vi "2D Animation Plot.vi"(4 "sample length":i32=1000, 6 "angle unit":u16(ring) items=["radians", "degrees"], 7 "reset":bool, 9 "Goal":cluster{"x":dbl, "y":dbl}={"x"=nan, "y"=nan}, 10 "2D Origin":cluster{"x":dbl, "y":dbl, "theta":dbl}, 11 "2D Translation":cluster{"x":dbl, "y":dbl, "theta":dbl}) -> (3 "Coordinate Frame":cluster{dbl[], dbl[]}[](graph))   [LabVIEW 2017]
uses:
  <vilib>/Analysis/baseanly.llb/Real A x B.vi
  LabVIEW Corke Toolkit/Functions/Position and Orientation/rvc Plot 2D Transform (scalar).vi
  <vilib>/ptbypt/NI_PtbyPt.lvlib
  <vilib>/Analysis/NI_AALBase.lvlib
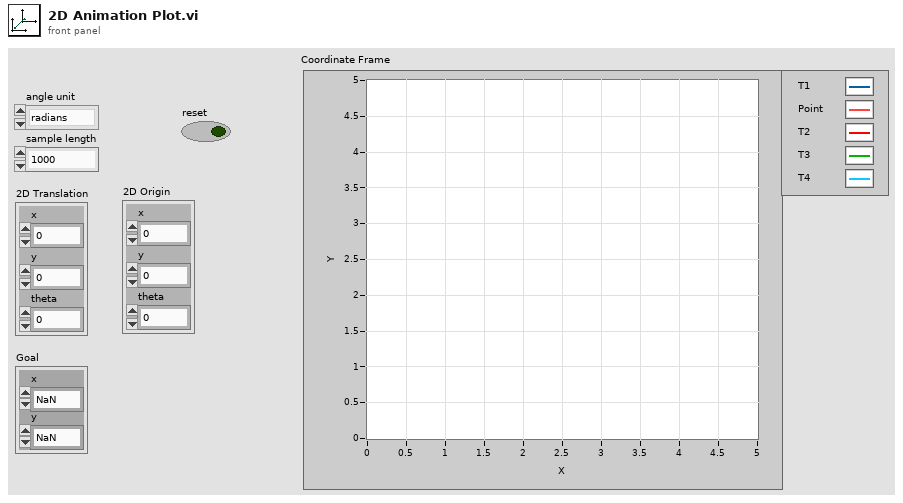
[diagram p1: front panel]
types:
  T1 = typedef "NI_Matrix.lvlib/RealMatrix.ctl" = dbl[][]
  T2 = cluster{"Current Queue":dbl[], "Current Queue":dbl[]}
  T3 = cluster{"Current Queue":dbl[], "Current Queue":dbl[]}[]
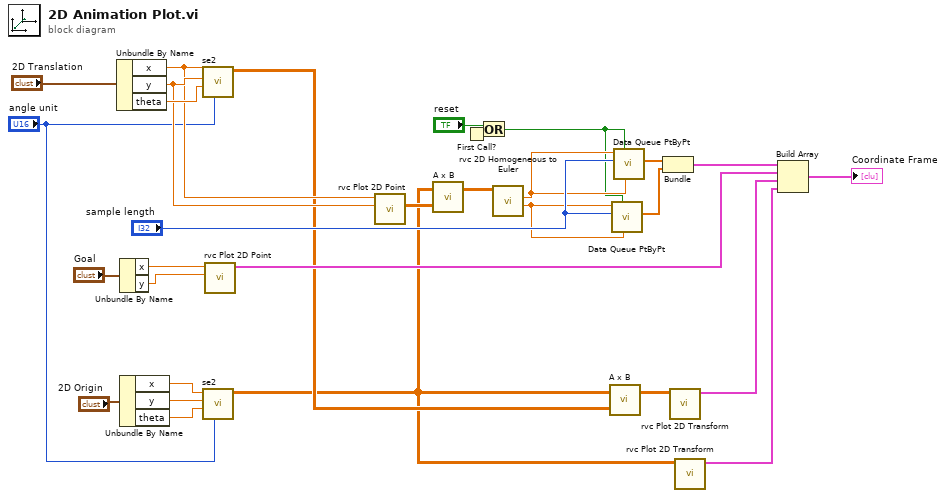
[diagram p0: block diagram]
diagram:
  n1 = Unbundle By Name("2D Translation") -> ("x"=w11:dbl, "y"=w12:dbl, "theta"=w25:dbl)
  n2 = Unbundle By Name("Goal") -> ("x"=w28:dbl, "y"=w27:dbl)
  n3 = Unbundle By Name("2D Origin") -> ("x"=w17:dbl, "y"=w16:dbl, "theta"=w15:dbl)
  n4 = call "se2.vi"("angle unit"="angle unit", "theta"=w25, "y"=w12, "x"=w11) -> ("T"=w10:dbl[][])  [unwired: 6 in, 1 out]
  n5 = call "se2.vi"("angle unit"="angle unit", "theta"=w15, "y"=w16, "x"=w17) -> ("T"=w8:dbl[][])  [unwired: 6 in, 1 out]
  n6 = call "rvc Plot 2D Point.vi"("Y"=w27, "X"=w28) -> ("XY Graph"=w30:cluster{dbl[], dbl[]})  [unwired: 8 in, 1 out]
  n7 = call "rvc Plot 2D Point.vi"("Y"=w12, "X"=w11) -> ("Column vector"=w9:dbl[][])  [unwired: 8 in, 1 out]
  n8 = call-poly <vilib>:"A x B.vi"("B"=w9, "A"=w8) -> ("A x B"=w13:T1)  [unwired: 1 out]
  n9 = First Call?() -> (First Call?: T/F=w5:bool)
  n10 = Or(x="reset", y=w5) -> (x .or. y?=w2:bool)
  n11 = call "rvc 2D Homogeneous to Euler.vi"("T"=w13) -> ("y"=w3:dbl, "x"=w4:dbl)  [unwired: 7 in, 2 out]
  n12 = call-poly <vilib>:"A x B.vi"("B"=w10, "A"=w8) -> ("A x B"=w14:T1)  [unwired: 1 out]
  n13 = call <vilib>:"Data Queue PtByPt.vi"("initial queue element"=w3, "initialize"=w2, "sample length"="sample length", "input data point"=w3) -> ("Current Queue"=w20:dbl[])  [unwired: 3 in, 4 out]
  n14 = call <vilib>:"Data Queue PtByPt.vi"("initial queue element"=w4, "initialize"=w2, "sample length"="sample length", "input data point"=w4) -> ("Current Queue"=w21:dbl[])  [unwired: 3 in, 4 out]
  n15 = Bundle("Current Queue"=w21, "Current Queue"=w20) -> (w19:T2)  [unwired: 1 in]
  n16 = call-poly "rvc Plot 2D Transform.vi"("T"=w14) -> ("XY Graph 2"=w24:cluster{dbl[], dbl[]})  [unwired: 9 in, 1 out]
  n17 = call-poly "rvc Plot 2D Transform.vi"("T"=w8) -> ("XY Graph 2"=w7:cluster{dbl[], dbl[]})  [unwired: 9 in, 1 out]
  n18 = Build Array(w19, w30, w24, w7) -> (→"Coordinate Frame":T3)
